vi "Control Panel - Close.vi"(8 "error in (no error)":errorcluster, 11 "Plugin Server in":refnum<class "Generic Plugin.lvclass">) -> (0 "error out":errorcluster, 3 "Plugin Server out":refnum<class "Generic Plugin.lvclass">)   [LabVIEW 2020, in "RxnRover.lvlib" / "Generic Plugin.lvclass"]
doc: "Initialize the Control Panel at the provided controller path. Forwards a stop message to the control panel process to signal that it should end."
uses:
  Generic Plugin.lvclass
  Generic Plugin.lvclass/Generic Plugin.ctl
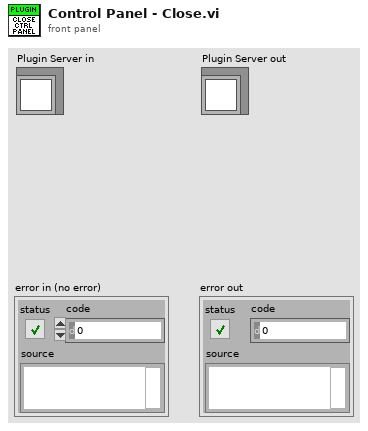
[diagram p1: front panel]
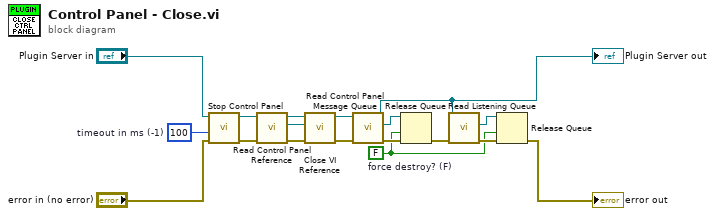
[diagram p0: block diagram]
diagram:
  w8 = 100  # timeout in ms (-1)
  w5 = FALSE  # force destroy? (F)
  n1 = call "Stop Control Panel.vi"("error in (no error)"="error in (no error)", "timeout in ms (-1)"=w8, "controller in"="Plugin Server in") -> ("error out"=w9:errorcluster, "controller out"=w10:refnum<class "Generic Plugin.lvclass">)  [unwired: 7 in]
  n2 = call "Read Control Panel Reference.vi"("error in (no error)"=w9, "controller in"=w10) -> ("error out"=w16:errorcluster, "Control Panel Reference"=w18:refnum<vi>, "controller out"=w17:refnum<class "Generic Plugin.lvclass">)  [unwired: 7 in]
  n3 = call "Close VI Reference.vi"("error in (no error)"=w16, "VI Refnum"=w18, "Plugin Server in"=w17) -> ("error out"=w14:errorcluster, "Plugin Server out"=w15:refnum<class "Generic Plugin.lvclass">)  [unwired: 6 in, 1 out]
  n4 = call "Read Control Panel Message Queue.vi"("error in (no error)"=w14, "Plugin Server in"=w15) -> ("error out"=w13:errorcluster, "Sending Queue"=w12:refnum<queue>, "Plugin Server out"=w1:refnum<class "Generic Plugin.lvclass">)  [unwired: 7 in]
  "Plugin Server out" <- w1
  n5 = Release Queue(queue=w12, force destroy? (F)=w5, error in (no error)=w13) -> (error out=w4:errorcluster)  [unwired: 2 out]
  n6 = call "Read Listening Queue.vi"("error in (no error)"=w4, "Generic Controller in"=w1) -> ("error out"=w7:errorcluster, "Listening Queue"=w6:refnum<queue>)  [unwired: 7 in, 1 out]
  n7 = Release Queue(queue=w6, force destroy? (F)=w5, error in (no error)=w7) -> (error out=→"error out":errorcluster)  [unwired: 2 out]
